vi "LV to Igor Graph (UI).vi"() -> ()   [LabVIEW 2019, in "Data.ITX.lvclass"]
uses:
  Data.ITX.lvclass
  Graph Utilities/graph_utilities.lvclass
panel:
  in  "Trace Names (XY Graph Only)":string[](array[string])=["first", "second", "third"]
  in  "X,Y,Z Scale Names":string[](array[string])=["X", "Y", "Z"]
  in  "Enum":enum16{"XY Graph", "Intensity Graph"}(ring)
  out "Tab":enum32{"XY Graph", "Intensity Graph"}(tab)
  in  "XY Graph":cluster{dbl[], dbl[]}[](graph)
  in  "Intensity Graph":dbl[][](graph)
  in  "Path":path=path "C:/temp"
  in  "Filename":string="testname"
  in  "open file in Igor?":bool
  # "<-- choose which graph you would like to save"
  # "Igor Syntax:\n\\S = superscript\n\\B = subscript\n\\M = normal\n\nExample:\nV\\MS\\B = \"V_S\""
  # "adjust offset and multiplier\nhere to make your graph look\ncorrect in Igor"
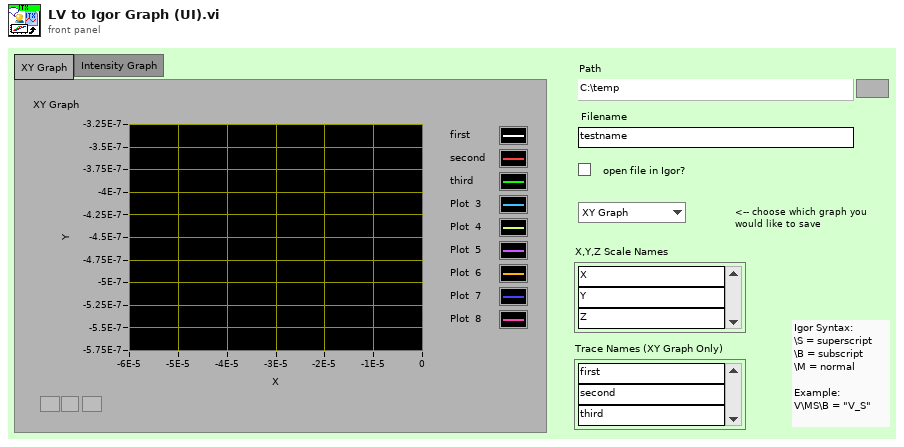
[diagram p1: front panel]
types:
  T1 = typedef "LVOffsetAndMultiplierTypeDef.ctl" = cluster{"Offset":dbl, "Multiplier":dbl}
  T2 = cluster{"Intensity Graph":dbl[][], "Array":dbl[], "Array":dbl[]}
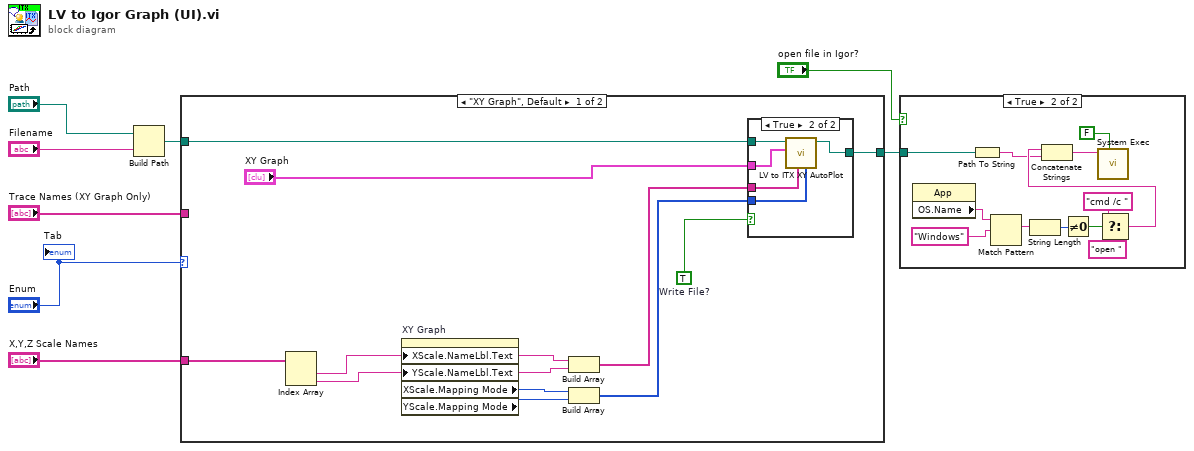
[diagram p0: block diagram]
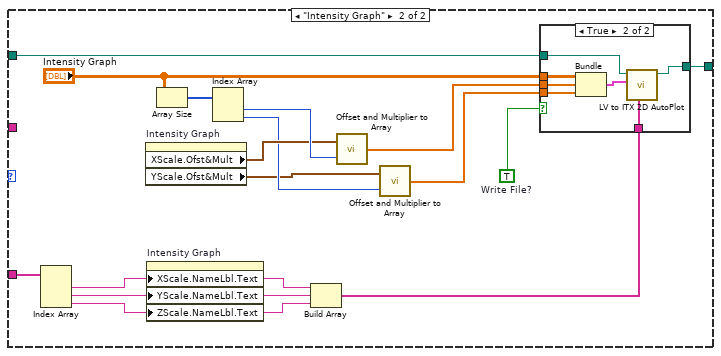
[diagram p4: hidden frame]
diagram:
  n1 = Build Path(base path="Path", name or relative path="Filename") -> (appended path=w2:path)
  n2 = case shown="\"XY Graph\", Default" "Enum" {
    tunnel: w2 -> [w19 w37]
    tunnel: [w18 w38] -> w8
    tunnel: "X,Y,Z Scale Names" -> [w13 w36]
    tunnel: "Trace Names (XY Graph Only)" -> [_ _]
    frame "XY Graph", Default {
      w10 = TRUE  # Write File?
      n3 = Index Array(array=w13) -> (element #1=w12:string, element #2=w11:string)  [unwired: 2 in]
      n4 = property on="XY Graph" class="XYGraph (strict)"("XScale.NameLbl.Text"=w12, "YScale.NameLbl.Text"=w11) -> ("XScale.Mapping Mode"=w16:u8, "YScale.Mapping Mode"=w15:u8)  [unwired: 2 in, 2 out]
      n5 = Build Array(w12, w11) -> (w17:string[])
      n6 = Build Array(w16, w15) -> (w14:u8[])
      n7 = case shown="True" w10 {
        tunnel: w19 -> [w20 w24]
        tunnel: "XY Graph" -> [_ w25]
        tunnel: [w20 w23] -> w18
        tunnel: w17 -> [_ w22]
        tunnel: w14 -> [_ w21]
        frame False {
        }
        frame True {
          n8 = call "LV to ITX XY AutoPlot.vi"("X,Y Log"=w21, "X,Y Labels"=w22, "XY-Data []"=w25, "path"=w24) -> ("file"=w23:path)  [unwired: 6 in, 1 out]
        }
      }
    }
    frame "Intensity Graph" {
      w32 = TRUE  # Write File?
      n9 = Index Array(array=w36) -> (element #1=w34:string, element #2=w35:string, element #3=w33:string)  [unwired: 3 in]
      n10 = property on="Intensity Graph" class="IntGraph (strict)"() -> ("XScale.Ofst&Mult"=w30:T1, "YScale.Ofst&Mult"=w27:T1)  [unwired: 2 in, 2 out]
      n11 = property on="Intensity Graph" class="IntGraph (strict)"("XScale.NameLbl.Text"=w34, "YScale.NameLbl.Text"=w35, "ZScale.NameLbl.Text"=w33) -> ()  [unwired: 2 in, 2 out]
      n12 = Array Size(array="Intensity Graph") -> (size(s)=w39:i32[])
      n13 = Index Array(array=w39) -> (element #1=w31:i32, element #2=w28:i32)  [unwired: 2 in]
      n14 = Build Array(w34, w35, w33) -> (w41:string[])
      n15 = call "Offset and Multiplier to Array.vi"("Size"=w31, "Offset and Multiplier"=w30) -> ("Array"=w29:dbl[])
      n16 = call "Offset and Multiplier to Array.vi"("Size"=w28, "Offset and Multiplier"=w27) -> ("Array"=w26:dbl[])
      n17 = case shown="True" w32 {
        tunnel: w41 -> [_ w44]
        tunnel: "Intensity Graph" -> [_ w49]
        tunnel: [w42 w45] -> w38
        tunnel: w37 -> [w42 w46]
        tunnel: w29 -> [_ w48]
        tunnel: w26 -> [_ w47]
        frame False {
        }
        frame True {
          n18 = Bundle("Intensity Graph"=w49, "Array"=w48, "Array"=w47) -> (w43:T2)  [unwired: 1 in]
          n19 = call "LV to ITX 2D AutoPlot.vi"("X,Y,Z Labels"=w44, "2D, X, Y (Cluster)"=w43, "path"=w46) -> ("file"=w45:path)  [unwired: 7 in, 1 out]
        }
      }
    }
  }
  n20 = case shown="True" "open file in Igor?" {
    tunnel: w8 -> [_ w53]
    frame False {
    }
    frame True {
      n21 = property class="App"() -> ("OS.Name"=w54:string)  [unwired: 2 in, 2 out]
      n22 = Path To String(path=w53) -> (string=w50:string)
      n23 = Match Pattern(string=w54, regular expression="Windows") -> (match substring=w60:string)  [unwired: 1 in, 3 out]
      n24 = String Length(string=w60) -> (length=w59:i32)
      n25 = Not Equal To 0?(x=w59) -> (x != 0?=w57:bool)
      n26 = Select(t="cmd /c ", s=w57, f="open ") -> (s? t:f=w52:string)
      n27 = Concatenate Strings(w52, w50) -> (w61:string)
      n28 = call <vilib>:"System Exec.vi"("wait until completion? (T)"=FALSE, "command line"=w61) -> ()  [unwired: 6 in, 4 out]
    }
  }
  "Tab" <- "Enum"
